vi "publisher.vi"() -> ()   [LabVIEW 2022 SP3]
panel:
  in  "stop":bool
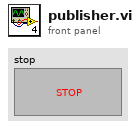
[diagram p1: front panel]
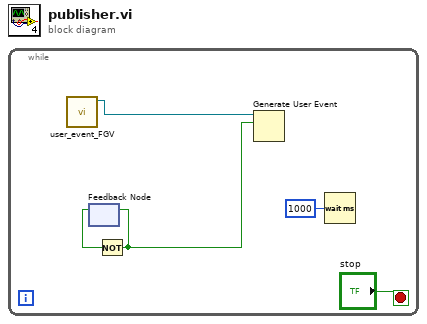
[diagram p0: block diagram]
diagram:
  n1 = while {
    stop <- "stop" stop-if-true
    n2 = call "user_event_FGV.vi"() -> ("bool"=w4:refnum<user-event>)  [unwired: 11 in]
    n3 = feedback #1() -> (w2:bool)  [unwired: 1 in]
    n4 = Not(x=w2) -> (.not. x?=w1:bool)
    n5 = feedback-in #1(w1) -> ()
    n6 = Generate User Event(user event=w4, event data cluster=w1) -> ()  [unwired: 2 in, 2 out]
    n7 = Wait (ms)(milliseconds to wait=u32 1000) -> ()  [unwired: 1 out]
  }
